vi "Write Key (String without quotation) workaround.vi"(6 "write raw string? (F)":bool, 7 "section":string, 8 "error in (no error)":errorcluster, 9 "value":string, 10 "key":string, 11 "refnum":T1) -> (0 "error out":errorcluster, 2 "found?":bool, 3 "refnum out":T1)   [LabVIEW 2010, in "NI_LVConfig.lvlib"]
doc: "Writes a value to a key in a specified section of the configuration data identified by <B>refnum</B>. This VI modifies data in memory. To write data to disk, use the Close Config Data VI. Wire data to the <B>value</B> input to determine the polymorphic instance to use or manually select the instance."
uses:
  <vilib>/Utility/config.llb/NI_LVConfig.lvlib
  <vilib>/Utility/config.llb/Config Data RefNum.ctl
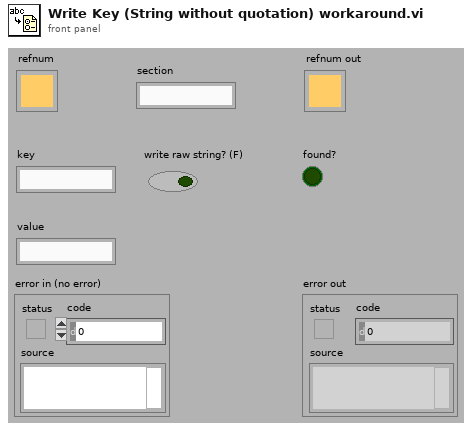
[diagram p1: front panel]
types:
  T1 = typedef "NI_LVConfig.lvlib/Config Data RefNum.ctl" = refnum<k1>
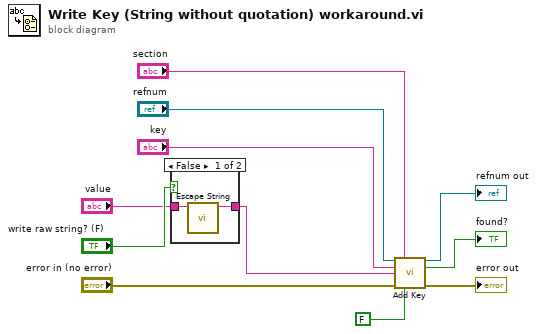
[diagram p0: block diagram]
diagram:
  n1 = case shown="False" "write raw string? (F)" {
    tunnel: "value" -> [w12 w14]
    tunnel: [w13 w14] -> w2
    frame False {
      n2 = call <vilib>:"Escape String.vi"("input"=w12) -> ("output"=w13:string)  [unwired: 10 in]
    }
    frame True {
    }
  }
  n3 = call <vilib>:"Add Key.vi"("refnum"="refnum", "section"="section", "key"="key", "value"=w2, "error in (no error)"="error in (no error)", "add comment"=FALSE) -> ("refnum out"=→"refnum out":T1, "key exists?"=→"found?":bool, "error out"=→"error out":errorcluster)  [unwired: 7 out]
